vi "run_auto_test.vi"(7 "Cluster":T2, 8 "error in (no error)":errorcluster) -> (0 "error out":errorcluster)   [LabVIEW 2019]
uses:
  core_dataRefCluster.ctl
  core_dataRef.ctl
  core_dataCluster.ctl
  instrument/instr_dataCluster.ctl
  gui/test_result_user_event1.ctl
  gui/test_results 1.ctl
  instrument/Instrument.lvclass
panel:
  in  "user_event_out":T1
  in  "modbusData":refnum<notifier>
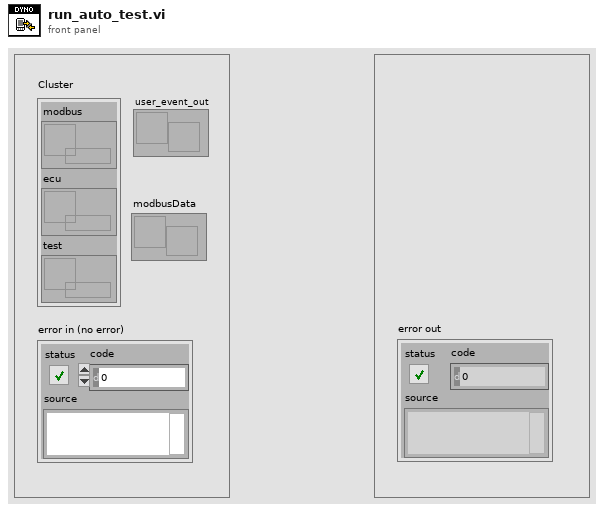
[diagram p1: front panel]
types:
  T1 = typedef "test_result_user_event1.ctl" = refnum<user-event>
  T2 = typedef "core_dataRefCluster.ctl" = cluster{"modbus":T3, "ecu":T3, "test":T3}
  T3 = typedef "core_dataRef.ctl" = refnum<queue>
  T4 = typedef "core_dataCluster.ctl" = cluster{"cmd":string, "data":variant}
  T5 = typedef "Instrument.lvclass/instr_dataCluster.ctl" = cluster{"电源电压 V":dbl, "电源电流A":dbl, "扭矩N/m":dbl, "速度r/M":dbl, "温度℃":dbl[], "流量计L/M":dbl[]}
  T6 = typedef "ecu_dataCluster.ctl" = cluster{"MCU_MotCtrlrSts":dbl, "MCU_MotTq":dbl, "MCU_MotBusU":dbl, "MCU_MotSpd":dbl, "MCU_MotBodyT":dbl, "MCU_MotBody_T":dbl, "MCU_MotCtrlrT":dbl, "MCU 状态":bool, "ErrMsg":i64}
  T7 = cluster{"电源电流A":dbl, bool, "phase current":dbl, bool}
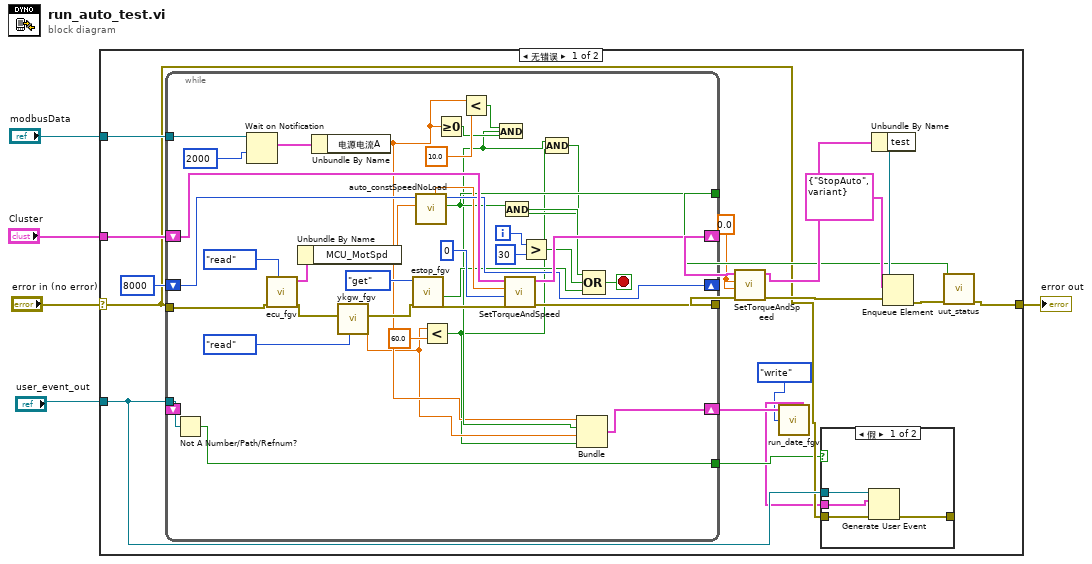
[diagram p0: block diagram]
diagram:
  n1 = case shown="无错误" "error in (no error)" {
    selector: "error in (no error)" -> [w10 w67]
    tunnel: "Cluster" -> [w24 _]
    tunnel: [w11 w67] -> w4
    tunnel: "modbusData" -> [w18 _]
    tunnel: "user_event_out" -> [w12 _]
    frame No Error {
      w14 = sgl 0.0 ("Torque")
      n2 = while {
        shift-right: [w65] -> w22
        shift-left: w24 -> [w66]
        shift-right: [w62] -> _
        shift-left: 8000 ("Speed") -> [w64]
        tunnel: [w45] -> w15
        tunnel: [w56] -> w19
        tunnel: w18 -> [w50]
        tunnel: w12 -> [w36]
        tunnel: w10 -> [w31]
        tunnel: [w29] -> w8
        shift-right: [w30] -> w9
        shift-left: _ -> [_]
        i -> [w61]
        stop <- w46 stop-if-true
        n3 = Not A Number/Path/Refnum?(number/path/refnum=w36) -> (NaN/Path/Refnum?=w29:bool)
        n4 = Wait on Notification(notifier=w50, timeout in ms (-1)=2000 ("超时毫秒(-1)")) -> (notification=w48:T5)  [unwired: 2 in, 3 out]
        n5 = call "ecu_fgv.vi"("mode"=enum16{"read", "write"}."read", "error in (no error)"=w31) -> ("error out"=w43:errorcluster, "data out"=w55:T6)  [unwired: 8 in]
        n6 = Unbundle By Name(w55) -> ("MCU_MotSpd"=w63:dbl)
        n7 = Unbundle By Name(w48) -> ("电源电流A"=w34:dbl)
        n8 = call "ykgw_fgv.vi"("mode"=enum16{"read", "write"}."read", "error in (no error)"=w43) -> ("phase current"=w33:dbl, "error out"=w42:errorcluster)  [unwired: 5 in, 3 out]
        n9 = call "estop_fgv.vi"("error in (no error)"=w42, "Enum"=enum16{"set", "get"}."get") -> ("error out"=w51:errorcluster, "indicator"=w52:bool)  [unwired: 8 in]
        n10 = call "auto_constSpeedNoLoad.vi"("speed"=w63, "Speed"=w64) -> ("Pass"=w45:bool, "Set speed"=w62:i32, "torque"=w58:sgl)  [unwired: 7 in]
        n11 = Less?(x=w33, y=60.0) -> (x < y?=w32:bool)
        n12 = Greater Or Equal To 0?(x=w34) -> (x >= 0?=w37:bool)
        n13 = Less?(x=w34, y=10.0) -> (x < y?=w38:bool)
        n14 = And(x=w38, y=w37) -> (x .and. y?=w35:bool)
        n15 = call "SetTorqueAndSpeed.vi"("error in (no error)"=w51, "Speed"=0, "Torque"=w58, "Cluster in"=w66) -> ("error out"=w56:errorcluster, "Cluster out"=w65:T2)  [unwired: 6 in]
        n16 = Greater?(x=w61, y=30) -> (0:w59:bool)
        n17 = Compound Arithmetic op=AND(w35, w32) -> (w40:bool)
        n18 = And(x=w45, y=w40) -> (x .and. y?=w47:bool)
        n19 = Bundle("电源电流A"=w34, w35, "phase current"=w33, w32) -> (w30:T7)  [unwired: 1 in]
        n20 = Compound Arithmetic op=OR(w47, w59, w52) -> (w46:bool)
      }
      n21 = call "SetTorqueAndSpeed.vi"("error in (no error)"=w19, "Speed"=w14, "Torque"=w14, "Cluster in"=w22) -> ("error out"=w13:errorcluster, "Cluster out"=w17:T2)  [unwired: 6 in]
      n22 = call "run_date_fgv .vi"("mode"=enum16{"read", "write"}."write", "DATE in"=w9) -> ("DATE OUT"=w7:cluster{"电源电流A":dbl, bool, "VI":dbl, bool})  [unwired: 1 in, 1 out]
      n23 = case shown="假" w8 {
        tunnel: [w28 _] -> _
        tunnel: w10 -> [w26 _]
        tunnel: w7 -> [w27 _]
        tunnel: w12 -> [w25 _]
        frame False {
          n24 = Generate User Event(user event=w25, event data cluster=w27, error in=w26) -> (error out=w28:errorcluster)  [unwired: 1 in, 1 out]
        }
        frame True {
        }
      }
      n25 = Unbundle By Name(w17) -> ("test"=w21:T3)
      n26 = Enqueue Element(queue=w21, element=T4 {"cmd"="StopAuto", "data"=variant}, error in (no error)=w13) -> (error out=w16:errorcluster)  [unwired: 1 in, 2 out]
      n27 = call "uut_status.vi"("error in (no error)"=w16, "status"=w15) -> ("error out"=w11:errorcluster)  [unwired: 9 in]
    }
    frame Error {
    }
  }
  "error out" <- w4
